vi "DC Voltmeter.vi"() -> ()   [LabVIEW 2015]
doc: "This VI turns the computer into a DC voltmeter. \nVspan for +/-5V:\n8-bit: 0.04V\n14-bit: 0.6mV\n16-bit: 0.2mV"
panel:
  in  "device name":tag="Dev1"
  out "error out":errorcluster
  out "Voltage":dbl format="%#.4g"
  in  "Stop":bool
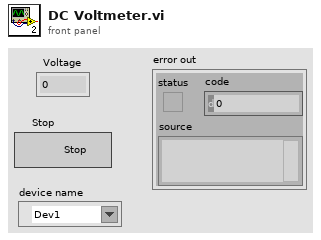
[diagram p1: front panel]
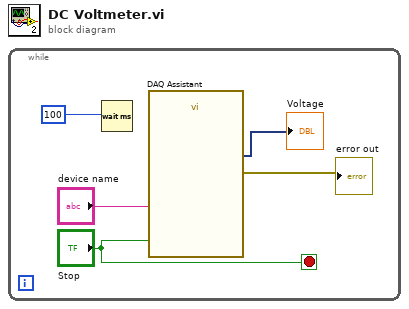
[diagram p0: block diagram]
diagram:
  n1 = while {
    stop <- "Stop" stop-if-true
    n2 = Wait (ms)(milliseconds to wait=u32 100) -> ()  [unwired: 1 out]
    n3 = call "DAQ Assistant"("stop (T)"="Stop", "device name"="device name") -> ("data"=→"Voltage":dynamicdata, "error out"=→"error out":errorcluster)  [unwired: 15 in, 1 out]
  }
